vi "liblinear_predict.vi"(8 "error in (no error)":errorcluster, 10 "x":T1[](array[typedef])=[{"index"=0, "value"=0.0}], 11 "liblinear_model":T2={"liblinear_parameter"={"solver_type"=0, "eps"=0.01, "C"=1.0, "weight_label"=[], "weight"=[], "p"=0.1}, "nr_class"=0, "nr_feature"=0, "w"=[], "label"=[], "bias"=0.0} {"liblinear_parameter"."solver_type" items=["L2R_LR"=0, "L2R_L2LOSS_SVC_DUAL"=1, "L2R_L2LOSS_SVC"=2, "L2R_L1LOSS_SVC_DUAL"=3, "MCSVM_CS"=4, "L1R_L2LOSS_SVC"=5, "L1R_LR"=6, "L2R_LR_DUAL"=7, "L2R_L2LOSS_SVR"=11, "L2R_L2LOSS_SVR_DUAL"=12, "L2R_L1LOSS_SVR_DUAL"=13]}) -> (0 "error out":errorcluster, 3 "predicted label":dbl)   [LabVIEW 2014]
uses:
  Controls/liblinear_model.ctl
  Controls/liblinear_parameter.ctl
  Controls/liblinear_solver.ctl
  Controls/liblinear_node.ctl
  <vilib>/oysstu/LVLibSVM/bin/x64/LVLibSVM.dll
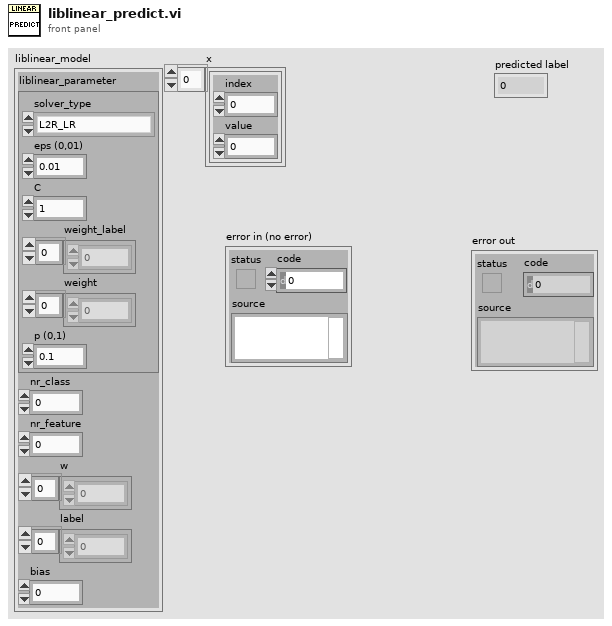
[diagram p1: front panel]
types:
  T1 = typedef "liblinear_node.ctl" = cluster{"index":i32, "value":dbl}
  T2 = typedef "liblinear_model.ctl" = cluster{"liblinear_parameter":T3, "nr_class":i32, "nr_feature":i32, "w":dbl[], "label":i32[], "bias":dbl}
  T3 = typedef "liblinear_parameter.ctl" = cluster{"solver_type":T4, "eps":dbl, "C":dbl, "weight_label":i32[], "weight":dbl[], "p":dbl}
  T4 = typedef "liblinear_solver.ctl" = u32
  T5 = typedef "liblinear_node_padded.ctl" = cluster{"index":i32, "padding":i32, "value":dbl}
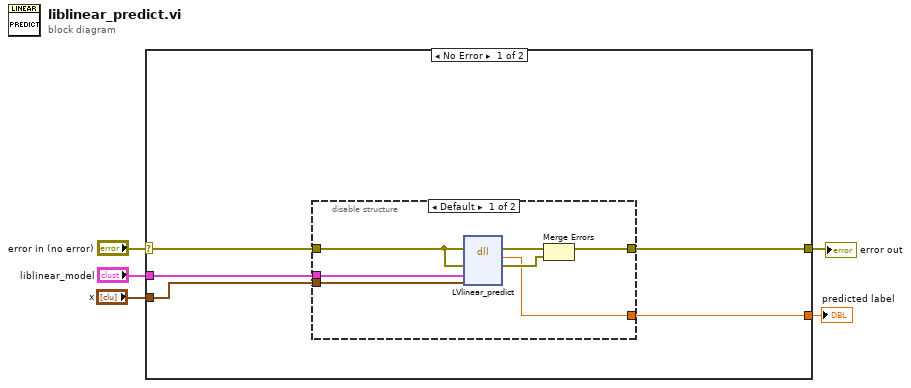
[diagram p0: block diagram]
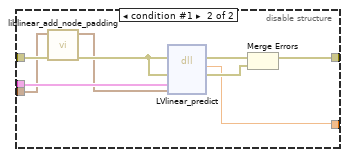
[diagram p2: hidden frame]
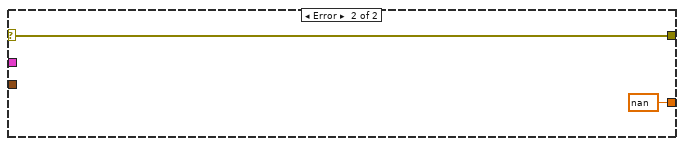
[diagram p3: hidden frame]
diagram:
  n1 = case shown="No Error" "error in (no error)" {
    selector: "error in (no error)" -> [w10 w28]
    tunnel: [w9 w28] -> w5
    tunnel: "liblinear_model" -> [w8 _]
    tunnel: "x" -> [w7 _]
    tunnel: [w6 nan ("predicted label")] -> w1
    frame No Error {
      n2 = disable-structure shown="Default" {
        disable-tunnel: w10 -> [w17 w22]
        disable-tunnel: [w15 w25] -> w9
        disable-tunnel: w8 -> [w13 w23]
        disable-tunnel: w7 -> [w12 w20]
        disable-tunnel: [w11 w18] -> w6
        frame condition #0 (active) {
          n3 = dll-call lib="C:/Program Files/National Instruments/LabVIEW 2014/vi.lib/oysstu/LVLibSVM/bin/x64/LVLibSVM.dll" fn="LVlinear_predict"(error in=w17, "lvErr"=w17, "model_in"=w13, "x_in"=w12) -> (error out=w16:errorcluster, "predicted label"=w11:dbl, "lvErr"=w14:errorcluster)  [unwired: 4 in, 1 out]
          n4 = Merge Errors(w16, w14) -> (w15:errorcluster)
        }
        frame condition #1 {
          n5 = call "liblinear_add_node_padding.vi"("error in (no error)"=w22, "Nodes"=w20) -> ("error out"=w21:errorcluster, "Padded nodes"=w19:T5[])  [unwired: 8 in]
          n6 = dll-call lib="C:/Program Files/National Instruments/LabVIEW 2014/vi.lib/oysstu/LVLibSVM/bin/x64/LVLibSVM.dll" fn="LVlinear_predict"(error in=w21, "lvErr"=w21, "model_in"=w23, "x_in"=w19) -> (error out=w26:errorcluster, "predicted label"=w18:dbl, "lvErr"=w24:errorcluster)  [unwired: 4 in, 1 out]
          n7 = Merge Errors(w26, w24) -> (w25:errorcluster)
        }
      }
    }
    frame Error {
    }
  }
  "error out" <- w5
  "predicted label" <- w1
